vi "BoolarraytoNumber.vi"() -> ()   [LabVIEW 2018]
panel:
  out "불리언 배열":bool[](array[boolean])
  out "숫자":u32
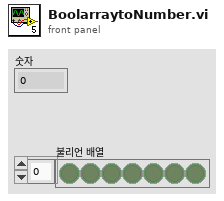
[diagram p1: front panel]
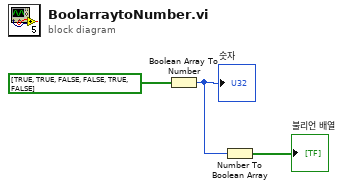
[diagram p0: block diagram]
diagram:
  n1 = Boolean Array To Number(Boolean array=bool[] [TRUE, TRUE, FALSE, FALSE, TRUE, FALSE]) -> (number=w2:u32)
  "숫자" <- w2
  n2 = Number To Boolean Array(number=w2) -> (Boolean array=→"불리언 배열":bool[])
